vi "sub_write_custom_pads.vi"(11 "input string":string) -> (3 "result string":string)   [LabVIEW 2020]
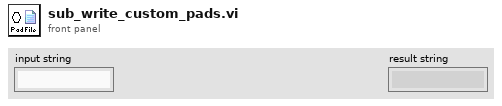
[diagram p1: front panel]
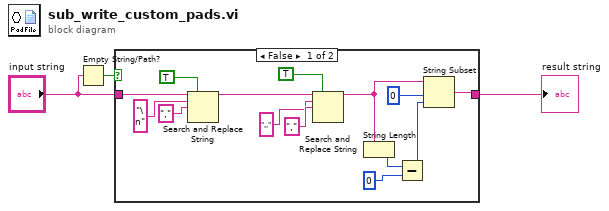
[diagram p0: block diagram]
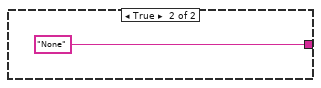
[diagram p2: hidden frame]
diagram:
  n1 = Empty String/Path?(string/path="input string") -> (empty?=w1:bool)
  n2 = case shown="False" w1 {
    tunnel: [w8 "None" ("result string")] -> w3
    tunnel: "input string" -> [w14 _]
    frame False {
      n3 = Search and Replace String(replace all?=TRUE ("replace all? (F)"), input string=w14, search string="\n", replace string="," ("replace string (\"\")")) -> (result string=w13:string)  [unwired: 4 in, 3 out]
      n4 = Search and Replace String(replace all?=TRUE ("replace all? (F)"), input string=w13, search string=",,", replace string="," ("replace string (\"\")")) -> (result string=w7:string)  [unwired: 4 in, 3 out]
      n5 = String Length(string=w7) -> (length=w9:i32)
      n6 = Subtract(x=w9, y=0) -> (x-y=w6:i32)
      n7 = String Subset(string=w7, offset (0)=0, length (rest)=w6) -> (substring=w8:string)
    }
    frame True {
    }
  }
  "result string" <- w3
